vi "Downsampler.vi"(2 "Input Array":dbl[](array[numeric]) format="%.2f", 3 "Averaging samples":i32=5) -> (0 "Downsampled Array":dbl[](array[numeric]) format="%.2f", 1 "Samples remaining":dbl[](array[numeric]) format="%.2f")   [LabVIEW 2021]
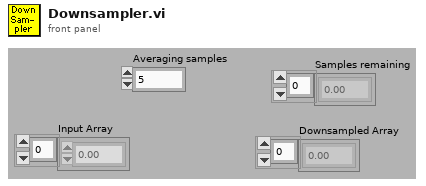
[diagram p1: front panel]
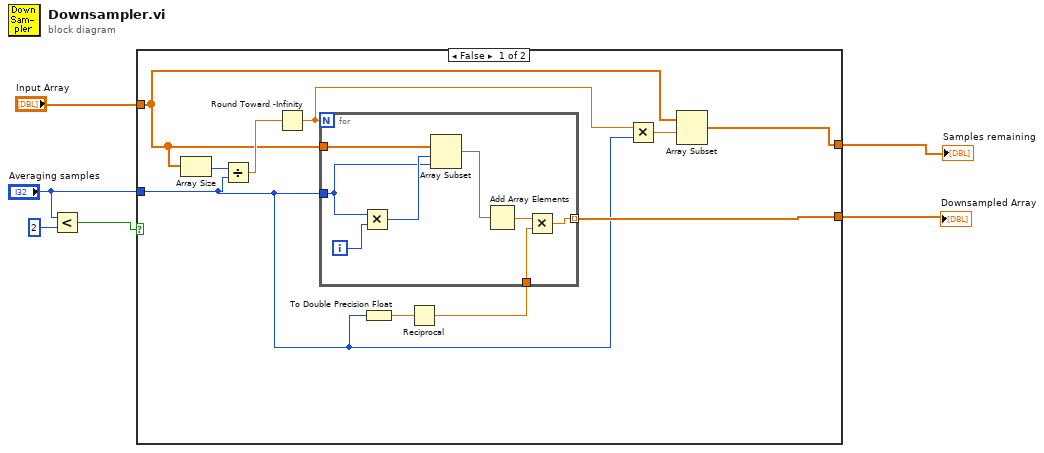
[diagram p0: block diagram]
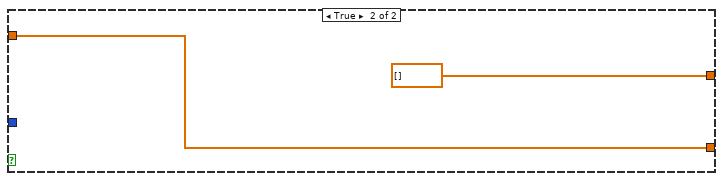
[diagram p2: hidden frame]
diagram:
  n1 = Less?(x="Averaging samples", y=2) -> (x < y?=w1:bool)
  n2 = case shown="False" w1 {
    tunnel: "Input Array" -> [w11 w26]
    tunnel: [w16 w26] -> w5
    tunnel: [w10 dbl[] [] ("Input Array")] -> w4
    tunnel: "Averaging samples" -> [w9 _]
    frame False {
      n3 = Array Size(array=w11) -> (size(s)=w15:i32)
      n4 = Divide(x=w15, y=w9) -> (x/y=w14:dbl)
      n5 = Round Toward -Infinity(1:w14) -> (0:w13:dbl)
      n6 = To Double Precision Float(number=w9) -> (double precision float=w8:dbl)
      n7 = Reciprocal(x=w8) -> (1/x=w7:dbl)
      n8 = for {
        N: w13 -> [_]
        tunnel: w9 -> [w21]
        tunnel: [w18] -> w16 mode=indexing
        tunnel: w11 -> [w24]
        tunnel: w7 -> [w17]
        i -> [w23]
        n9 = Multiply(x=w21, y=w23) -> (x*y=w22:i32)
        n10 = Array Subset(array=w24, index=w22, length=w21) -> (w20:dbl[])
        n11 = Add Array Elements(numeric array=w20) -> (sum=w19:dbl)
        n12 = Multiply(x=w19, y=w17) -> (x*y=w18:dbl)
      }
      n13 = Multiply(x=w13, y=w9) -> (x*y=w12:dbl)
      n14 = Array Subset(array=w11, index=w12) -> (w10:dbl[])  [unwired: 1 in]
    }
    frame True {
    }
  }
  "Downsampled Array" <- w5
  "Samples remaining" <- w4
